vi "overlay sides on room image.vi"(8 "error in (no error)":errorcluster, 10 "image data in":T1, 11 "Room in":refnum<class "Room.lvclass">) -> (0 "error out":errorcluster, 2 "image data  out":T1, 3 "Room out":refnum<class "Room.lvclass">)   [LabVIEW 2016, in "Room.lvclass"]
uses:
  Room.lvclass
  <vilib>/picture/picture.llb/imagedata.ctl
  Room.lvclass/Room.ctl
  MapSite/MapSite.lvclass
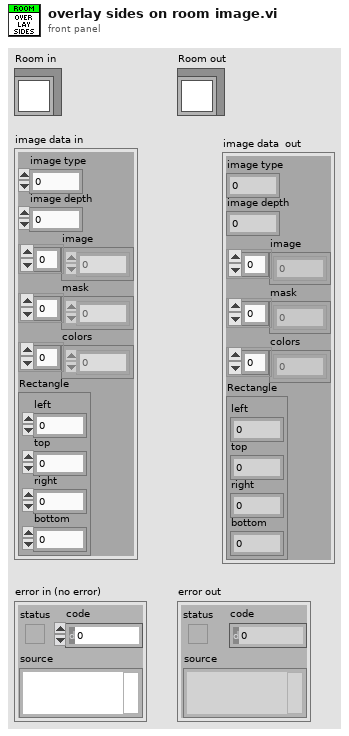
[diagram p1: front panel]
types:
  T1 = typedef "imagedata.ctl" = cluster{"image type":i32, "image depth":i32, "image":u8[], "mask":u8[], "colors":u32[], "Rectangle":cluster{"left":i16, "top":i16, "right":i16, "bottom":i16}}
  T2 = cluster{"left":i16, "top":i16, "right":i16, "bottom":i16}
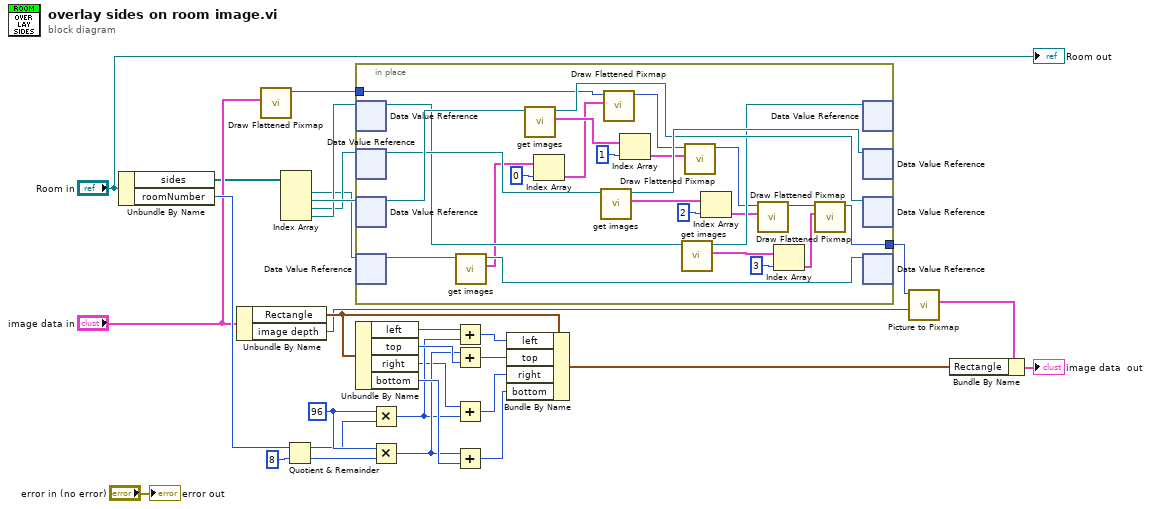
[diagram p0: block diagram]
diagram:
  w30 = 96 ("y")
  n1 = Unbundle By Name("Room in") -> ("sides"=w4:refnum<data-value>[], "roomNumber"=w13:i32)
  n2 = Unbundle By Name("image data in") -> ("Rectangle"=w19:T2, "image depth"=w12:i32)
  n3 = call <vilib>:"Draw Flattened Pixmap.vi"("image data"="image data in") -> ("new picture"=w9:picture)  [unwired: 8 in]
  n4 = Index Array(array=w4) -> (element #1=w5:refnum<data-value>, element #2=w8:refnum<data-value>, element #3=w6:refnum<data-value>, element #4=w7:refnum<data-value>)  [unwired: 4 in]
  n5 = Quotient & Remainder(x=w13, y=8) -> (x-y*floor(x/y)=w15:i32, floor(x/y)=w22:i32)
  n6 = in-place {
    in-place-border: w9 -> [w38]
    in-place-border: [w31] -> w10
    n7 = in-place-dvr #1(w7) -> (w49:refnum<class "MapSite.lvclass">)  [unwired: 1 out]
    n8 = in-place-dvr #2(w6) -> (w52:refnum<class "MapSite.lvclass">)  [unwired: 1 out]
    n9 = in-place-dvr #3(w8) -> (w54:refnum<class "MapSite.lvclass">)  [unwired: 1 out]
    n10 = in-place-dvr #4(w5) -> (w55:refnum<class "MapSite.lvclass">)  [unwired: 1 out]
    n11 = call-dynamic "get images.vi"("MapSite in"=w55) -> ("images"=w47:T1[], "MapSite out"=w53:refnum<class "MapSite.lvclass">)  [unwired: 8 in, 1 out]
    n12 = call-dynamic "get images.vi"("MapSite in"=w54) -> ("images"=w46:T1[], "MapSite out"=w50:refnum<class "MapSite.lvclass">)  [unwired: 8 in, 1 out]
    n13 = Index Array(array=w47, index=0) -> (element=w39:T1)
    n14 = call-dynamic "get images.vi"("MapSite in"=w52) -> ("images"=w45:T1[], "MapSite out"=w51:refnum<class "MapSite.lvclass">)  [unwired: 8 in, 1 out]
    n15 = call <vilib>:"Draw Flattened Pixmap.vi"("image data"=w39, "picture"=w38) -> ("new picture"=w37:picture)  [unwired: 7 in]
    n16 = Index Array(array=w46, index=1) -> (element=w34:T1)
    n17 = call-dynamic "get images.vi"("MapSite in"=w49) -> ("images"=w44:T1[], "MapSite out"=w48:refnum<class "MapSite.lvclass">)  [unwired: 8 in, 1 out]
    n18 = call <vilib>:"Draw Flattened Pixmap.vi"("image data"=w34, "picture"=w37) -> ("new picture"=w36:picture)  [unwired: 7 in]
    n19 = Index Array(array=w45, index=2) -> (element=w33:T1)
    n20 = call <vilib>:"Draw Flattened Pixmap.vi"("image data"=w33, "picture"=w36) -> ("new picture"=w35:picture)  [unwired: 7 in]
    n21 = Index Array(array=w44, index=3) -> (element=w32:T1)
    n22 = call <vilib>:"Draw Flattened Pixmap.vi"("image data"=w32, "picture"=w35) -> ("new picture"=w31:picture)  [unwired: 7 in]
    n23 = in-place-dvr #1(w48) -> ()  [unwired: 2 out]
    n24 = in-place-dvr #2(w51) -> ()  [unwired: 2 out]
    n25 = in-place-dvr #3(w50) -> ()  [unwired: 2 out]
    n26 = in-place-dvr #4(w53) -> ()  [unwired: 2 out]
  }
  n27 = Unbundle By Name(w19) -> ("left"=w16:i16, "top"=w24:i16, "right"=w17:i16, "bottom"=w25:i16)
  n28 = Multiply(x=w30, y=w15) -> (x*y=w18:i32)
  n29 = Multiply(x=w30, y=w22) -> (x*y=w23:i32)
  n30 = Add(x=w16, y=w18) -> (x+y=w20:i32)
  n31 = Add(x=w23, y=w24) -> (x+y=w26:i32)
  n32 = Add(x=w17, y=w18) -> (x+y=w21:i32)
  n33 = Add(x=w23, y=w25) -> (x+y=w27:i32)
  n34 = Bundle By Name(cluster=w19, "left"=w20, "top"=w26, "right"=w21, "bottom"=w27) -> (w29:T2)
  n35 = call <vilib>:"Picture to Pixmap.vi"("depth"=w12, "picture"=w10) -> ("image data"=w28:T1)  [unwired: 8 in, 1 out]
  n36 = Bundle By Name(cluster=w28, "Rectangle"=w29) -> (→"image data  out":T1)
  "error out" <- "error in (no error)"
  "Room out" <- "Room in"
